vi "GetParam.vi"(8 "error in (no error)":errorcluster caption="entrée d'erreur (pas d'erreur)", 11 "Classification.lvclass":refnum<class "Classification.lvclass">) -> (0 "error out":errorcluster caption="sortie d'erreur", 2 "make_classification":T1={"n_samples"=100, "n_features"=20, "n_informative"=2, "n_redundant"=2, "n_repeated"=0, "n_classes"=2, "n_clusters_per_class"=2, "weights"=[], "flip_y"=0.01, "class_sep"=1.0, "hypercube"=TRUE, "shift"=[], "scale"=[], "shuffle"=TRUE, "random_state"=-1, "Returns"="X"} {"random_state" min=-1; "n_clusters_per_class" min=1; "n_classes" min=1; "n_features" min=1; "n_samples" min=1}, 3 "Classification.lvclass":refnum<class "Classification.lvclass">)   [LabVIEW 2020, in "Classification.lvclass"]
doc: "Get Parameters"
uses:
  Classification.lvclass
  Classification.lvclass/Classification.ctl
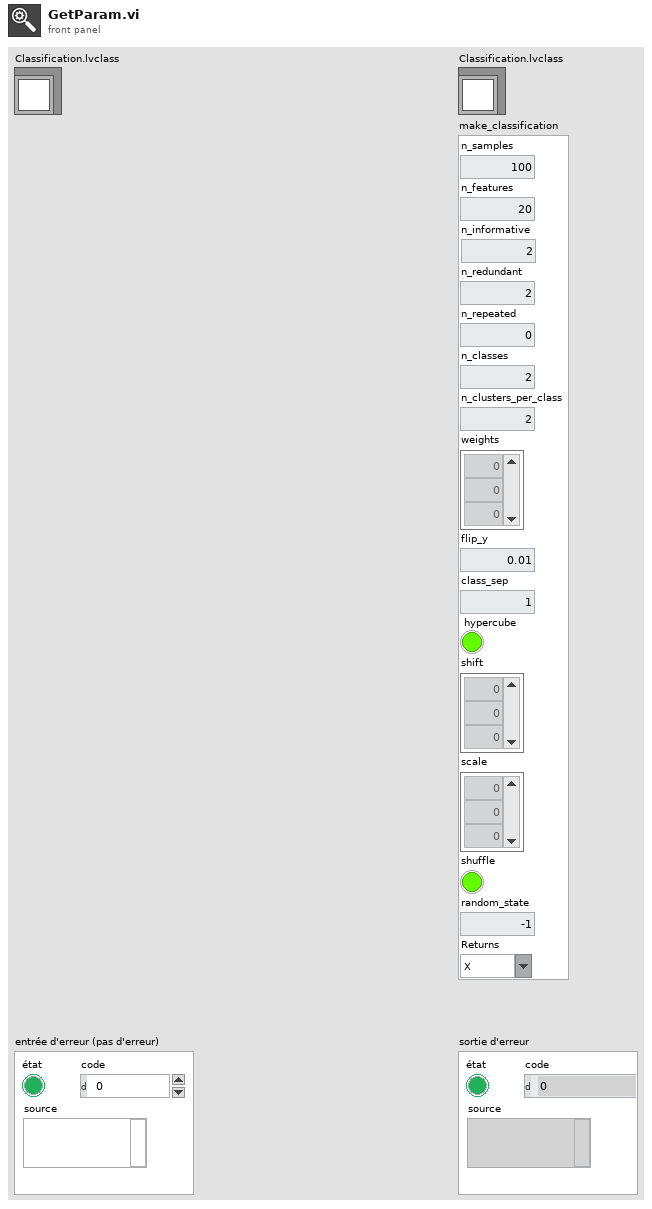
[diagram p1: front panel]
types:
  T1 = cluster{"n_samples":u32, "n_features":u32, "n_informative":i32, "n_redundant":i32, "n_repeated":i32, "n_classes":u32, "n_clusters_per_class":u32, "weights":i32[], "flip_y":dbl, "class_sep":dbl, "hypercube":bool, "shift":dbl[], "scale":dbl[], "shuffle":bool, "random_state":i32, "Returns":string}
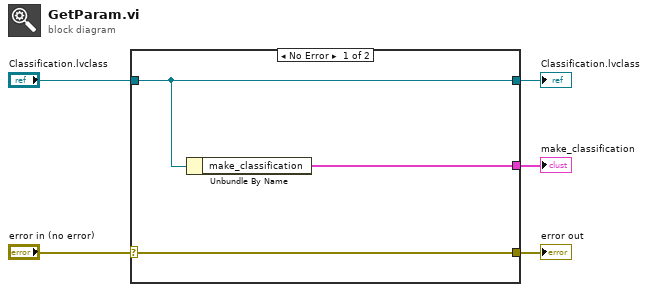
[diagram p0: block diagram]
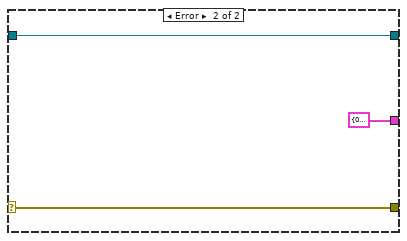
[diagram p2: hidden frame]
diagram:
  n1 = case shown="No Error" "error in (no error)" {
    selector: "error in (no error)" -> [w8 w10]
    tunnel: [w8 w10] -> w4
    tunnel: [w7 w11] -> w2
    tunnel: "Classification.lvclass" -> [w7 w11]
    tunnel: [w6 T1 {"n_samples"=0, "n_features"=0, "n_informative"=0, "n_redundant"=0, "n_repeated"=0, "n_classes"=0, "n_clusters_per_class"=0, "weights"=[], "flip_y"=0.0, "class_sep"=0.0, "hypercube"=FALSE, "shift"=[], "scale"=[], "shuffle"=FALSE, "random_state"=0, "Returns"=""} ("make_classification")] -> w1
    frame No Error {
      n2 = Unbundle By Name(w7) -> ("make_classification"=w6:T1)
    }
    frame Error {
    }
  }
  "error out" <- w4
  "Classification.lvclass" <- w2
  "make_classification" <- w1
